vi "Load Properties.vi"(8 "error in":errorcluster caption="错误输入（无错误）", 10 "Properties":string[](array[string]), 11 "PanelRootNode 输入":refnum<class "PanelRootNode.lvclass"> caption="DNL_LabVIEW Object in") -> (0 "error out":errorcluster caption="错误输出", 3 "PanelRootNode 输出":refnum<class "PanelRootNode.lvclass"> caption="DNL_LabVIEW Object out")   [LabVIEW 2016, in "PanelRootNode.lvclass"]
uses:
  PanelRootNode.lvclass
  C:/Users/CL/Desktop/ZcDAQprj0811/ZcDAQprj/Modules/DAQ-Display/PanelSplitToolkit/PanelDataNode/PanelDataNode.lvclass
  PanelDataNode/PanelDataNode.lvclass
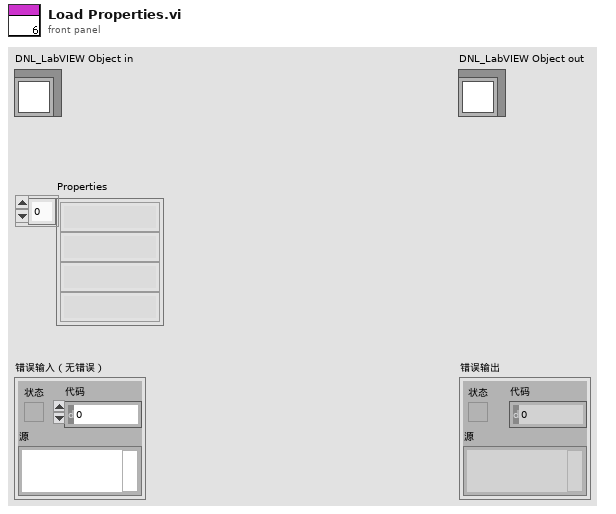
[diagram p1: front panel]
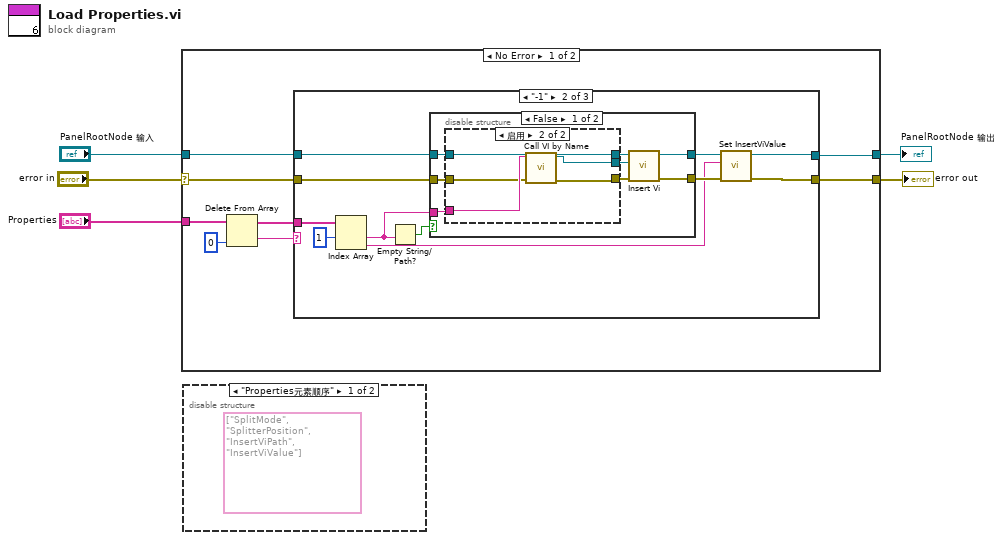
[diagram p0: block diagram]
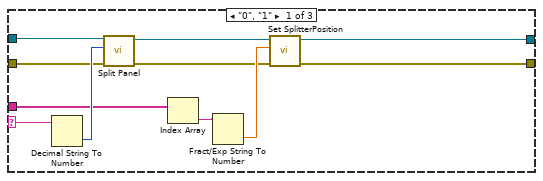
[diagram p3: hidden frame]
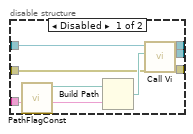
[diagram p4: hidden frame]
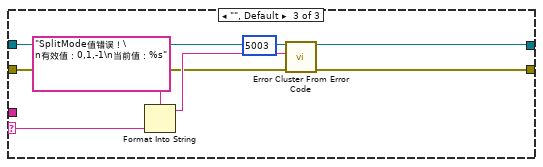
[diagram p6: hidden frame]
diagram:
  n1 = case shown="No Error" "error in" {
    selector: "error in" -> [w6 w67]
    tunnel: [w7 w67] -> w4
    tunnel: [w8 w66] -> w2
    tunnel: "PanelRootNode 输入" -> [w10 w66]
    tunnel: "Properties" -> [w13 _]
    frame No Error {
      n2 = Delete From Array(array=w13, index=0 ("索引")) -> (deleted portion=w9:string, array with subset deleted=w11:string[])  [unwired: 1 in]
      n3 = case shown="\"-1\"" w9 {
        selector: w9 -> [w24 _ w64]
        tunnel: w11 -> [w19 w35 _]
        tunnel: w10 -> [w23 w32 w65]
        tunnel: [w20 w29 w65] -> w8
        tunnel: [w15 w27 w61] -> w7
        tunnel: w6 -> [w14 w25 w60]
        frame "0", "1" {
          n4 = Decimal String To Number(string=w24) -> (number=w22:i32)  [unwired: 2 in, 1 out]
          n5 = call-dynamic "Split Panel.vi"("error in"=w14, "Split Mode"=w22, "PanelDataNode 输入"=w23) -> ("error out"=w16:errorcluster, "PanelDataNode 输出"=w21:refnum<class "PanelRootNode.lvclass">)  [unwired: 6 in, 1 out]
          n6 = Index Array(array=w19) -> (element=w18:string)  [unwired: 1 in]
          n7 = Fract/Exp String To Number(string=w18) -> (number=w17:dbl)  [unwired: 3 in, 1 out]
          n8 = call "Set SplitterPosition.vi"("error in (no error)"=w16, "Position(relative)"=w17, "PanelDataNode 输入"=w21) -> ("error out"=w15:errorcluster, "PanelDataNode 输出"=w20:refnum<class "PanelRootNode.lvclass">)  [unwired: 7 in]
        }
        frame "-1" {
          n9 = Index Array(array=w35, index #1=1 ("索引")) -> (element #1=w31:string, element #2=w26:string)  [unwired: 1 in]
          n10 = Empty String/Path?(string/path=w31) -> (empty?=w33:bool)
          n11 = case shown="False" w33 {
            tunnel: [w43 w58] -> w30
            tunnel: [w42 w57] -> w28
            tunnel: w31 -> [w41 _]
            tunnel: w32 -> [w40 w58]
            tunnel: w25 -> [w36 w57]
            frame False {
              n12 = disable-structure shown="启用" {
                disable-tunnel: w41 -> [w51 w55]
                disable-tunnel: w40 -> [w50 w56]
                disable-tunnel: [w49 w56] -> w39
                disable-tunnel: [w47 w52] -> w38
                disable-tunnel: [w46 w53] -> w37
                disable-tunnel: w36 -> [w45 w54]
                frame Disabled {
                  n13 = call "PathFlagConst.vi"() -> ("路径"=w44:path)  [unwired: 11 in]
                  n14 = Build Path(base path=w44, name or relative path=w51) -> (appended path=w48:path)
                  n15 = call-dynamic "Call Vi.vi"("error in (no error)"=w45, "Vi Path"=w48, "PanelDataNode 输入"=w50) -> ("error out"=w46:errorcluster, "VI*"=w47:refnum<vi>, "PanelDataNode 输出"=w49:refnum<class "PanelRootNode.lvclass">)  [unwired: 6 in]
                }
                frame Enabled {
                  n16 = call "Call VI by Name.vi"("error in"=w54, "VI Name"=w55) -> ("错误输出"=w53:errorcluster, "Dynamic vi reference out"=w52:refnum<vi>)  [unwired: 7 in, 1 out]
                }
              }
              n17 = call-dynamic "Insert Vi.vi"("error in (no error)"=w37, "VI*"=w38, "PanelDataNode 输入"=w39) -> ("error out"=w42:errorcluster, "PanelDataNode 输出"=w43:refnum<class "PanelRootNode.lvclass">)  [unwired: 7 in]
            }
            frame True {
            }
          }
          n18 = call-dynamic "Set InsertViValue.vi"("error in (no error)"=w28, "ViValue"=w26, "PanelDataNode 输入"=w30) -> ("error out"=w27:errorcluster, "PanelDataNode 输出"=w29:refnum<class "PanelRootNode.lvclass">)  [unwired: 7 in]
        }
        frame "", Default {
          n19 = Format Into String(format string="SplitMode值错误！\n有效值：0,1,-1\n当前值：%s" ("格式字符串"), w64) -> (resulting string=w62:string)  [unwired: 2 in, 1 out]
          n20 = call <vilib>:"Error Cluster From Error Code.vi"("error in (no error)"=w60, "error message (\"\")"=w62, "error code (0)"=5003) -> ("error out"=w61:errorcluster)  [unwired: 6 in]
        }
      }
    }
    frame Error {
    }
  }
  "error out" <- w4
  "PanelRootNode 输出" <- w2
  n21 = disable-structure shown="\"Properties元素顺序\"" {
    frame condition #0 {
      (unwired) string[] ["SplitMode", "SplitterPosition", "InsertViPath", "InsertViValue"]
    }
    frame condition #1 (active) {
    }
  }
